vi "lab_xyzp.vi"() -> ()   [LabVIEW 2023]
panel:
  out "x":bool
  in  "p_in":bool
  in  "z_in":bool
  in  "y_in":bool
  in  "x_in":bool
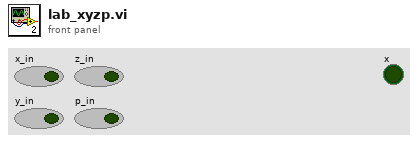
[diagram p1: front panel]
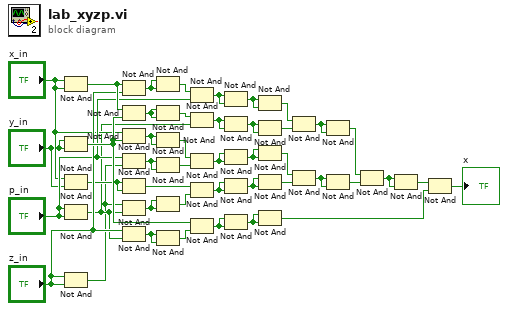
[diagram p0: block diagram]
diagram:
  n1 = Not And(1:"x_in", 2:"x_in") -> (0:w37:bool)
  n2 = Not And(1:"y_in", 2:"y_in") -> (0:w33:bool)
  n3 = Not And(1:"y_in", 2:"x_in") -> (0:w26:bool)
  n4 = Not And(1:"p_in", 2:"p_in") -> (0:w22:bool)
  n5 = Not And(1:"z_in", 2:"z_in") -> (0:w21:bool)
  n6 = Not And(1:"z_in", 2:w37) -> (0:w41:bool)
  n7 = Not And(1:w33, 2:w37) -> (0:w38:bool)
  n8 = Not And(1:w33, 2:"x_in") -> (0:w34:bool)
  n9 = Not And(1:w21, 2:"p_in") -> (0:w32:bool)
  n10 = Not And(1:w26, 2:w26) -> (0:w19:bool)
  n11 = Not And(1:w22, 2:w21) -> (0:w23:bool)
  n12 = Not And(1:w22, 2:"z_in") -> (0:w43:bool)
  n13 = Not And(1:w41, 2:w41) -> (0:w39:bool)
  n14 = Not And(1:w38, 2:w38) -> (0:w35:bool)
  n15 = Not And(1:w34, 2:w34) -> (0:w28:bool)
  n16 = Not And(1:w32, 2:w32) -> (0:w27:bool)
  n17 = Not And(1:w23, 2:w23) -> (0:w18:bool)
  n18 = Not And(1:w43, 2:w43) -> (0:w42:bool)
  n19 = Not And(1:"p_in", 2:w39) -> (0:w40:bool)
  n20 = Not And(1:w22, 2:w35) -> (0:w36:bool)
  n21 = Not And(1:w27, 2:w28) -> (0:w29:bool)
  n22 = Not And(1:w18, 2:w19) -> (0:w20:bool)
  n23 = Not And(1:w42, 2:w33) -> (0:w44:bool)
  n24 = Not And(1:w40, 2:w40) -> (0:w15:bool)
  n25 = Not And(1:w36, 2:w36) -> (0:w14:bool)
  n26 = Not And(1:w29, 2:w29) -> (0:w11:bool)
  n27 = Not And(1:w20, 2:w20) -> (0:w10:bool)
  n28 = Not And(1:w44, 2:w44) -> (0:w2:bool)
  n29 = Not And(1:w15, 2:w15) -> (0:w17:bool)
  n30 = Not And(1:w14, 2:w14) -> (0:w16:bool)
  n31 = Not And(1:w11, 2:w11) -> (0:w13:bool)
  n32 = Not And(1:w10, 2:w10) -> (0:w12:bool)
  n33 = Not And(1:w2, 2:w2) -> (0:w4:bool)
  n34 = Not And(1:w16, 2:w17) -> (0:w7:bool)
  n35 = Not And(1:w12, 2:w13) -> (0:w6:bool)
  n36 = Not And(1:w7, 2:w7) -> (0:w9:bool)
  n37 = Not And(1:w6, 2:w6) -> (0:w8:bool)
  n38 = Not And(1:w8, 2:w9) -> (0:w3:bool)
  n39 = Not And(1:w3, 2:w3) -> (0:w5:bool)
  n40 = Not And(1:w4, 2:w5) -> (0:→"x":bool)
